vi "Afterpulsing.vi"() -> ()   [LabVIEW 2012]
panel:
  in  "number":i32(ring) items=["Channel3"=2, "Channel2"=1, "Channel1"=0]
  in  "AP ON":bool
  out "Start time":u32
  out "XY Graph":cluster{"Y":dbl[], "Y":dbl[]}[](graph)
  out "Aftrerpulsing":dbl
  out "Single Count Channel3":dbl format="%#_3p"
  out "Single Count Channel2":dbl format="%#_3p"
  in  "Channel3 Pulse Front":string(combo)
  in  "Channel2 Pulse Front":string(combo)
  out "Single Count Channel1":dbl format="%#_3p"
  out "Exposition time (ms)":i64
  out "Measurement index":i64
  out "Start OK":bool
  in  "Exit":bool
  in  "Channel3 Threshold Voltage (mV)":i32
  in  "Channel2 Threshold Voltage (mV)":i32
  in  "Channel1 Pulse Front":string(combo)
  in  "Channel1 Threshold Voltage (mV)":i32 min=0 max=5000 step=10
  in  "Exposition Time (ms)":i64
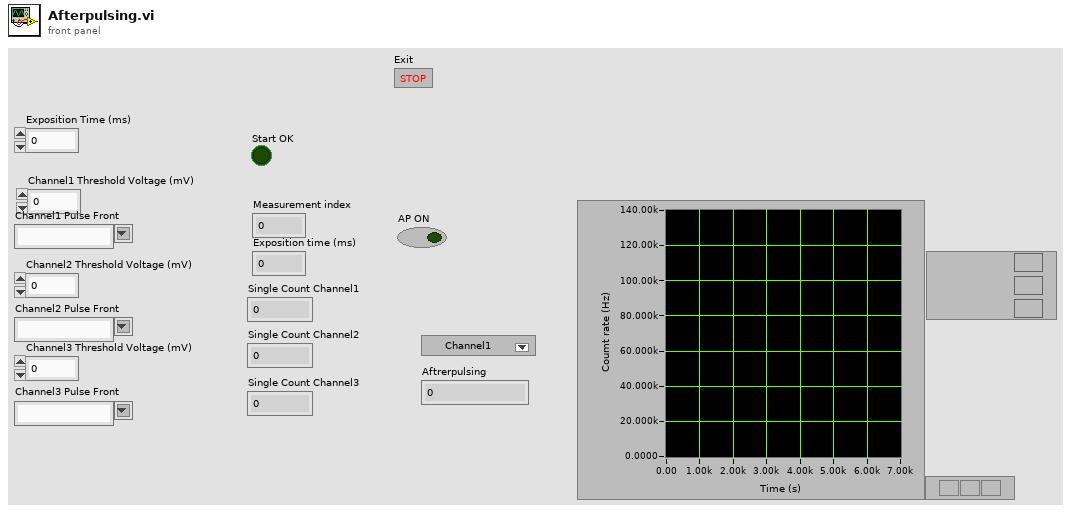
[diagram p1: front panel]
types:
  T1 = cluster{"Channel1":bool, "Channel2":bool, "Channel3":bool, "Channel4":bool}
  T2 = cluster{"[0]":i64, "Channel1 Threshold Voltage (mV)":i32, "Channel1 Pulse Front":string, "Channel2 Threshold Voltage (mV)":i32, "Channel2 Pulse Front":string, "Channel3 Threshold Voltage (mV)":i32, "Channel3 Pulse Front ":string, "Channel4 Threshold Voltage (mV)":i32, "Channel4 Pulse Front ":string, "Single Count Enable":cluster{"Channel1":bool, "Channel2":bool, "Channel3":bool, "Channel4":bool}, "Single Count Max":i32, "Sum Count Enable":cluster{"Channel1":bool, "Channel2":bool, "Channel3":bool, "Channel4":bool}, "Sum Count Max":i32, "Start-Stop1 Multyplex":cluster{"Stop Channel":string, "Start Channel":string}, "Stop Delay 1 (ns)":i16, "Window Length 1 (ns)":i32, "Window Offset 1 (ns) ":i32, "Conditional Correlation 1":string, "Histogram Bin 1":string, "Histogram Start 1 (ns) ":i32, "Start-Stop2 Multyplex ":cluster{"Stop Channel":string, "Start Channel":string}, "Stop Delay 2 (ns)":i16, "Window Length 2 (ns) ":i32, "Window Offset 2 (ns) ":i32, "Conditional Correlation 2":string, "Histogram Bin 2":string, "Histogram Start 2 (ns)  ":i32, "Start-Stop3 Multyplex":cluster{"Stop Channel":string, "Start Channel":string}, "Stop Delay 3 (ns)":i16, "Window Length 3 (ns) ":i32, "Window Offset 3 (ns) ":i32, "Conditional Correlation 3":string, "Histogram Bin 3":string, "Histogram Start 3 (ns) ":i32, "Start-Stop4 Multyplex":cluster{"Stop Channel":string, "Start Channel":string}, "Stop Delay 4 (ns)":i16, "Window Length 4 (ns)  ":i32, "Window Offset 4 (ns) ":i32, "Conditional Correlation 4":string, "Histogram Bin 4":string, "Histogram Start 4 (ns)  ":i32, "Coincidence Count Enable":cluster{"Start-Stop1":bool, "Start-Stop2":bool, "Start-Stop3":bool, "Start-Stop4":bool}, "Coincidence Count Max":i32, "Coincidence Sum Enable":cluster{"Start-Stop1":bool, "Start-Stop2":bool, "Start-Stop3":bool, "Start-Stop4":bool}, "Coincidence Sum Max":i32, "Output Channel Enable":cluster{"Channel1":bool, "Channel2":bool, "Channel3":bool, "Channel4":bool}, "Output Channel Inversion":cluster{"Channel1":bool, "Channel2":bool, "Channel3":bool, "Channel4":bool, "Output":bool}}
  T3 = cluster{"Going":bool, "Iinterrupted":bool, "Timer stop":bool, "Single count stop Ch1":bool, "Single count stop Ch2":bool, "Single count stop Ch3":bool, "Single count stop Ch4":bool, "Sum count stop":bool, "Coincidence count stop SS1":bool, "Coincidence count stop SS2":bool, "Coincidence count stop SS3":bool, "Coincidence count stop SS4":bool, "Coincidence sum count stop":bool, "Reserved":bool, "Correlator is not initialised":bool, "Internal error":bool}
  T4 = cluster{"Measurement index":i64, "Exposition time (ms)":i64, "Single Count Channel1":i64, "Single Count Channel2":i64, "Single Count Channel3":i64, "Single Count Channel4":i64, "Sum Single Count":i64, "Coincidence Count SS1":i64, "Coincidence Count SS2":i64, "Coincidence Count SS4":i64, "Coincidence Count SS5":i64, "Sum Coincidence Count":i64}
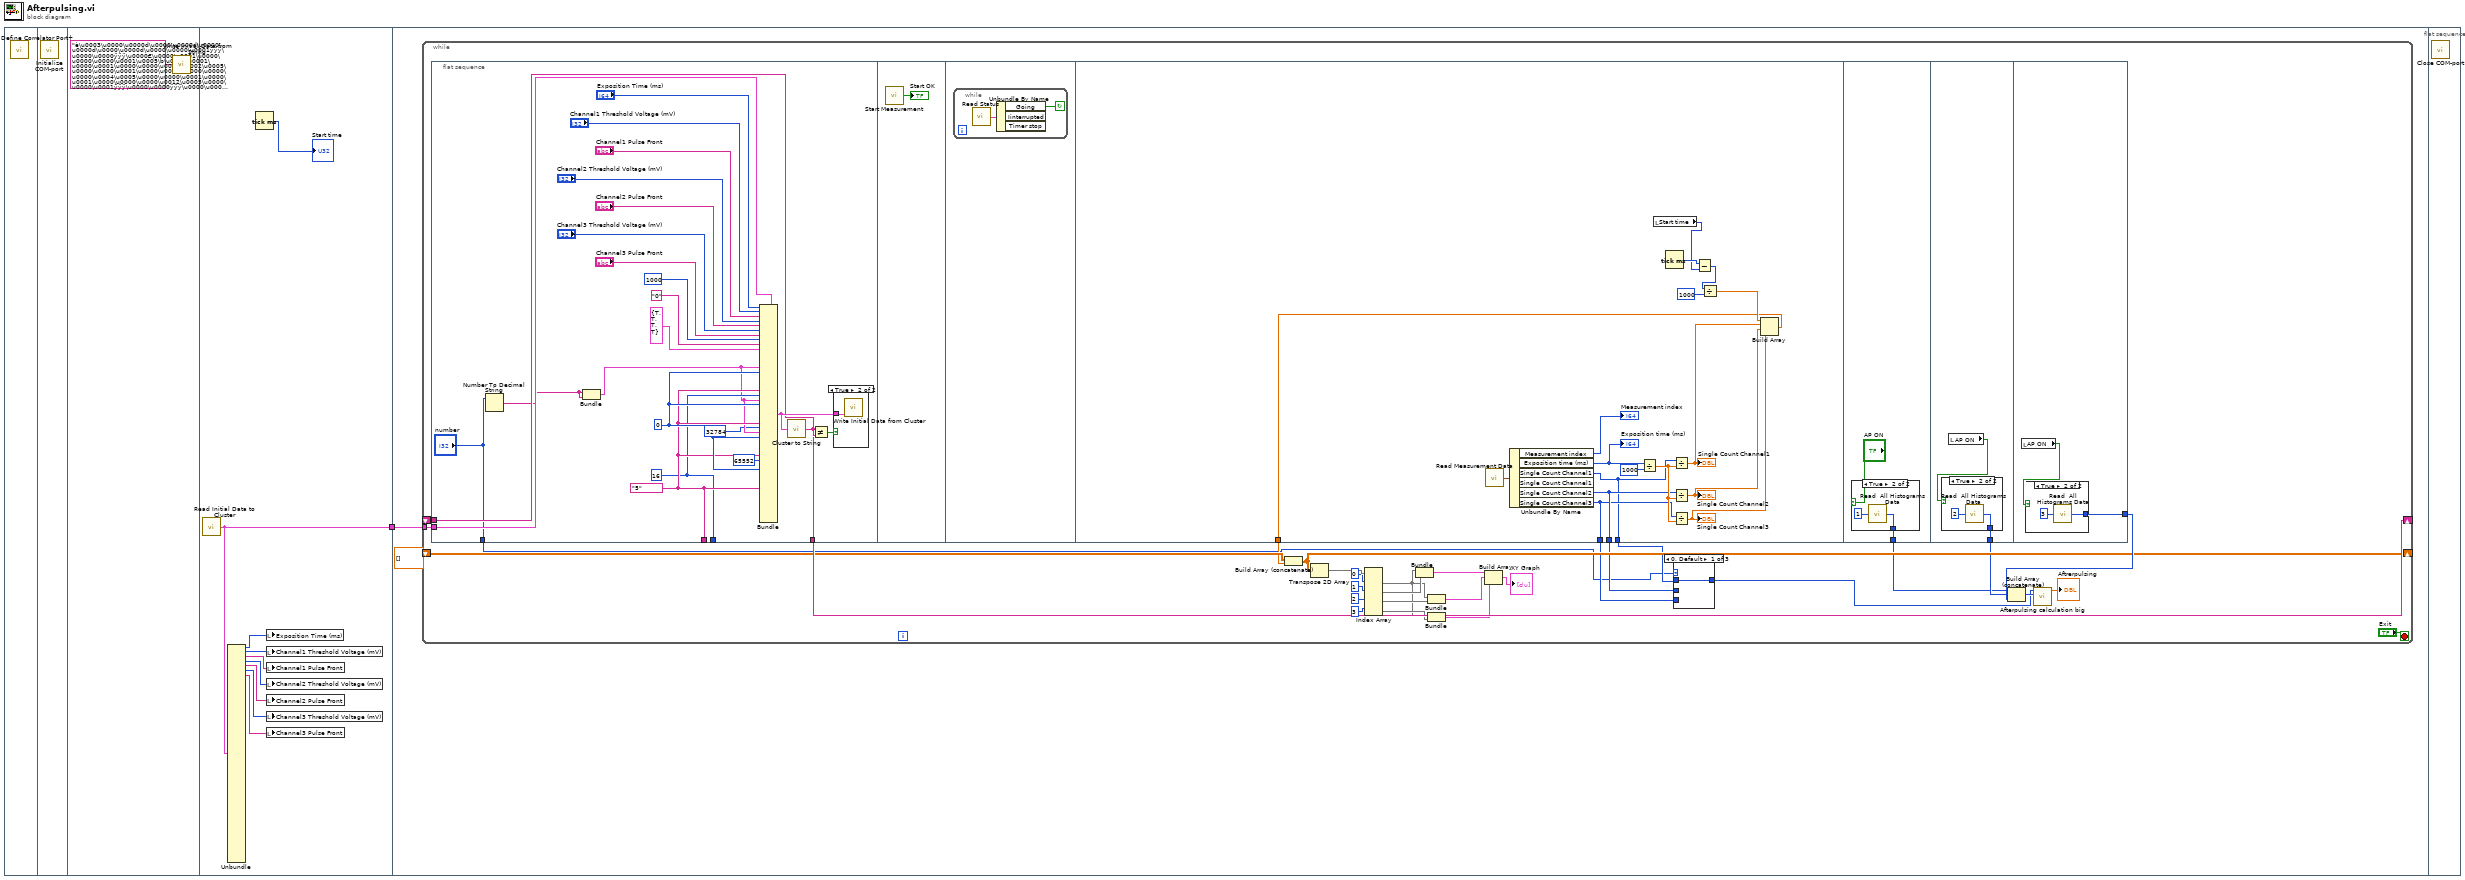
[diagram p0: block diagram]
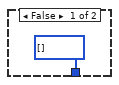
[diagram p5: hidden frame]
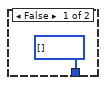
[diagram p6: hidden frame]
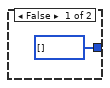
[diagram p7: hidden frame]
diagram:
  n1 = flat-sequence {
    tunnel: [w11] -> w1
    tunnel: w1 -> [w13]
    frame #0 {
      n2 = call "Define Correlator Port+.vi"() -> ()  [unwired: 3 in]
    }
    frame #1 {
      n3 = call "Initialize COM-port.vi"() -> ()  [unwired: 4 in]
    }
    frame #2 {
      n4 = call "Write Initial Data from String.vi"("Data"="è\u0003\u0000\u0000d\u0000\u0000d\u0000\u0000d\u0000\u0000d\u0000\u0000\u0001ÿÿÿ\u0000\u0000ÿÿÿ\u0000€\u0000\u0001\u0000\u0000\u0000\u0001\u0005\b\u0000\u0001\u0000\u0001\u0000\u0000\u0000\u0002\u0005\u0000\u0000\u0001\u0000\u0001\u0000\u0000\u0000\u0004\u0005\u0000\u0000\u0001\u0000\u0001\u0000\u0000\u0000\u0012\u0005\u0000\u0000\u0001ÿÿÿ\u0000\u0000ÿÿÿ\u0000\u0000\u0000" ("string")) -> ()  [unwired: 1 out]
    }
    frame #3 {
      n5 = call "Read Initial Data to Cluster.vi"() -> ("Correlator Initial Data 2"=w11:T2)  [unwired: 2 in]
      n6 = Unbundle(w11) -> ("[0]"=w10:i64, "Channel1 Threshold Voltage (mV)"=w9:i32, "Channel1 Pulse Front"=w8:string, "Channel2 Threshold Voltage (mV)"=w7:i32, "Channel2 Pulse Front"=w5:string, "Channel3 Threshold Voltage (mV)"=w6:i32, "Channel3 Pulse Front"=w4:string)  [unwired: 40 out]
      n7 = Tick Count (ms)() -> (millisecond timer value=→"Start time":u32)
      n8 = local write "Exposition Time (ms)"(w10) -> ()
      n9 = local write "Channel1 Threshold Voltage (mV)"(w9) -> ()
      n10 = local write "Channel1 Pulse Front"(w8) -> ()
      n11 = local write "Channel2 Threshold Voltage (mV)"(w7) -> ()
      n12 = local write "Channel2 Pulse Front"(w5) -> ()
      n13 = local write "Channel3 Threshold Voltage (mV)"(w6) -> ()
      n14 = local write "Channel3 Pulse Front"(w4) -> ()
    }
    frame #4 {
      n15 = while {
        tunnel: w13 -> [w42]
        shift-right: [w41] -> _
        shift-left: _ -> [w40]
        shift-right: [w22] -> _
        shift-left: dbl[][] [] -> [w24]
        stop <- "Exit" stop-if-true
        n16 = flat-sequence {
          tunnel: w42 -> [w64]
          tunnel: [w52] -> _
          tunnel: [w54] -> _
          tunnel: [w53] -> w41
          tunnel: w40 -> [w56]
          tunnel: ["number"] -> w14
          tunnel: [w85] -> w16
          tunnel: [w84] -> w15
          tunnel: [w83] -> w17
          tunnel: [w74] -> w23
          tunnel: [w92] -> w19
          tunnel: [w97] -> w20
          tunnel: [w102] -> w38
          frame #0 {
            w52 = 16 ("Histogram Start 1 (ns)")
            w54 = "5" ("Histogram Bin")
            w58 = i16 0 ("Stop Delay1  (ns)")
            n17 = Number To Decimal String(number="number") -> (decimal integer string=w51:string)  [unwired: 1 in]
            n18 = Bundle(w51, w51) -> (w50:cluster{string, string})  [unwired: 1 in]
            n19 = Bundle(cluster=w64, "[0]"="Exposition Time (ms)", "Channel1 Threshold Voltage (mV)"="Channel1 Threshold Voltage (mV)", "Channel1 Pulse Front"="Channel1 Pulse Front", "Channel2 Threshold Voltage (mV)"="Channel2 Threshold Voltage (mV)", "Channel2 Pulse Front"="Channel2 Pulse Front", "Channel3 Threshold Voltage (mV)"="Channel3 Threshold Voltage (mV)", "Channel3 Pulse Front"="Channel3 Pulse Front", "Channel4 Threshold Voltage (mV)"=1000, "Channel4 Pulse Front"="0", "Single Count Enable"=T1 {"Channel1"=TRUE, "Channel2"=TRUE, "Channel3"=TRUE, "Channel4"=TRUE}, "Start-Stop1 Multyplex"=w50, "Stop Delay 1 (ns)"=w58, "Histogram Bin 1"=w54, "Histogram Start 1 (ns)"=w52, "Start-Stop2 Multyplex"=w50, "Stop Delay 2 (ns)"=w58, "Histogram Bin 2"=w54, "Histogram Start 2 (ns)"=32784, "Start-Stop3 Multyplex"=w50, "Stop Delay 3 (ns)"=w58, "Histogram Bin 3"=w54, "Histogram Start 3 (ns)"=65552, "Stop Delay 4 (ns)"=w58, "Histogram Bin 4"=w54) -> (w57:T2)  [unwired: 23 in]
            n20 = call "Cluster to String.vi"("Correlator Initial Data"=w57) -> ("string"=w53:string)
            n21 = Not Equal?(x=w53, y=w56) -> (x != y?=w55:bool)
            n22 = case shown="True" w55 {
              tunnel: w57 -> [_ w70]
              frame False {
              }
              frame True {
                n23 = call "Write Initial Data from Cluster.vi"("Correlator Initial Data"=w70) -> ()  [unwired: 2 in, 1 out]
              }
            }
          }
          frame #1 {
            n24 = call "Start Measurement.vi"() -> ("Start OK"=→"Start OK":bool)  [unwired: 2 in]
          }
          frame #2 {
            n25 = while {
              stop <- w72 continue-if-true
              n26 = call "Read Status.vi"() -> ("Status Data"=w73:T3)  [unwired: 2 in]
              n27 = Unbundle By Name(w73) -> ("Going"=w72:bool)  [unwired: 2 out]
            }
          }
          frame #3 {
            n28 = call "Read Measurement Data.vi"() -> ("Measurement Data"=w89:T4)  [unwired: 3 in]
            n29 = Unbundle By Name(w89) -> ("Measurement index"=→"Measurement index":i64, "Exposition time (ms)"=w88:i64, "Single Count Channel1"=w83:i64, "Single Count Channel2"=w85:i64, "Single Count Channel3"=w84:i64)  [unwired: 1 out]
            "Exposition time (ms)" <- w88
            n30 = Divide(x=w88, y=1000) -> (x/y=w86:dbl)
            n31 = local read "Start time"() -> (w81:u32)
            n32 = Tick Count (ms)() -> (millisecond timer value=w82:u32)
            n33 = Divide(x=w83, y=w86) -> (x/y=w77:dbl)
            "Single Count Channel1" <- w77
            n34 = Divide(x=w85, y=w86) -> (x/y=w76:dbl)
            "Single Count Channel2" <- w76
            n35 = Divide(x=w84, y=w86) -> (x/y=w75:dbl)
            "Single Count Channel3" <- w75
            n36 = Subtract(x=w82, y=w81) -> (x-y=w80:u32)
            n37 = Divide(x=w80, y=u32 1000) -> (x/y=w78:dbl)
            n38 = Build Array(w78, w77, w76, w75) -> (w74:dbl[])
          }
          frame #4 {
            n39 = case shown="True" "AP ON" {
              tunnel: [i64[] [] ("Array") w94] -> w92
              frame False {
              }
              frame True {
                n40 = call "Read  All Histograms Data.vi"("Start-Stop#"=i8 1) -> ("Array"=w94:i64[])
              }
            }
          }
          frame #5 {
            n41 = local read "AP ON"() -> (w96:bool)
            n42 = case shown="True" w96 {
              tunnel: [i64[] [] ("Array") w99] -> w97
              frame False {
              }
              frame True {
                n43 = call "Read  All Histograms Data.vi"("Start-Stop#"=i8 2) -> ("Array"=w99:i64[])
              }
            }
          }
          frame #6 {
            n44 = local read "AP ON"() -> (w101:bool)
            n45 = case shown="True" w101 {
              tunnel: [i64[] [] ("Array") w104] -> w102
              frame False {
              }
              frame True {
                n46 = call "Read  All Histograms Data.vi"("Start-Stop#"=i8 3) -> ("Array"=w104:i64[])
              }
            }
          }
        }
        n47 = Build Array (concatenate)(w24, w23) -> (w22:dbl[][])
        n48 = Transpose 2D Array(2D array=w22) -> (transposed array=w37:dbl[][])
        n49 = Index Array(array=w37, index (row) #1=0 ("index (row)"), index (row) #2=1 ("disabled index (col)"), index (row) #3=2 ("index (row)"), index (row) #4=3 ("index (row)")) -> (element #1=w29:dbl[], element #2=w32:dbl[], element #3=w31:dbl[], element #4=w30:dbl[])  [unwired: 4 in]
        n50 = Bundle(w29, w32) -> (w28:cluster{dbl[], dbl[]})  [unwired: 1 in]
        n51 = Bundle(w29, w31) -> (w27:cluster{dbl[], dbl[]})  [unwired: 1 in]
        n52 = Bundle(w29, w30) -> (w26:cluster{dbl[], dbl[]})  [unwired: 1 in]
        n53 = Build Array(w28, w27, w26) -> (→"XY Graph":cluster{dbl[], dbl[]}[])
        n54 = case shown="0, Default" w14 {
          tunnel: [w44 w45 w46] -> w18
          tunnel: w17 -> [w44 _ _]
          tunnel: w16 -> [_ w45 _]
          tunnel: w15 -> [_ _ w46]
          frame 0, Default {
          }
          frame 1 {
          }
          frame 2 {
          }
        }
        n55 = Build Array (concatenate)(w19, w20, w38) -> (w21:i64[])
        n56 = call "Afterpulsing calculation big.vi"("Histogram with 128 ns bin"=w21, "Total counts"=w18) -> ("Afterpulsing probability (%)"=→"Aftrerpulsing":dbl)  [unwired: 9 in]
      }
    }
    frame #5 {
      n57 = call "Close COM-port.vi"() -> ()  [unwired: 4 in]
    }
  }
